vi "ScanPos.vi"(8 "DimScan":cluster{"Start":dbl, "Stop":dbl, "Steps":u32}, 11 "ScanPos":i32) -> (3 "Pos":dbl)   [LabVIEW 2013]
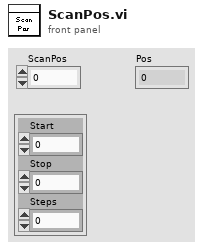
[diagram p1: front panel]
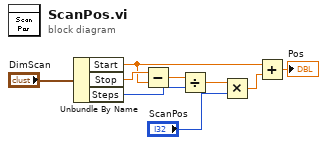
[diagram p0: block diagram]
diagram:
  n1 = Unbundle By Name("DimScan") -> ("Start"=w3:dbl, "Stop"=w8:dbl, "Steps"=w6:u32)
  n2 = Subtract(x=w8, y=w3) -> (x-y=w7:dbl)
  n3 = Divide(x=w7, y=w6) -> (x/y=w5:dbl)
  n4 = Multiply(x=w5, y="ScanPos") -> (x*y=w2:dbl)
  n5 = Add(x=w3, y=w2) -> (x+y=→"Pos":dbl)
